vi "getPosInfo.vi"(11 "UI_DataIn":T2={"controlTabState"=[], "pathToSTLFiles"=path "", "availableObjs"=[], "objectNames"=[], "addedObjs"=[], "selectedObj"={"Name"="", "objectFiles"=[], "center"={"X"=0.0, "Y"=0.0, "Z"=0.0}, "extent"={"X"=0.0, "Y"=0.0, "Z"=0.0}, "allowedMotion"=enum."XY", "mountOn"=enum."yArm", "Movements"=[], "extraInfo"=[], "hasPOI?"=FALSE, "POI"={"X"=0.0, "Y"=0.0, "Z"=0.0}, "posOffset"={"X"=0.0, "Y"=0.0, "Z"=0.0}, "referenceNum"=refnum}, "3DPictureObjRef"=refnum, "yPOI_Home"={"X"=0.0, "Y"=0.0, "Z"=0.0}, "yPOI_Current"={"X"=0.0, "Y"=0.0, "Z"=0.0}, "yPOI_Added?"=FALSE, "homePos_Offset"={"X"=0.0, "Y"=0.0, "Z"=0.0}, "breadBoardOriginOffset"={"X"=25.4, "Y"=12.7, "Z"=12.7}, "XYtranslateObjControls"=[], "ZtranslateObjControls"=[], "pBot_controls"=[], "pBot_VISA"="", "commandLog"="", "pBotConnected?"=FALSE, "pBot_currentEEPROMsettings"="", "realTimeInfoControls"=[], "pBot_tempSensor1"=0.0, "pBot_tempSensor2"=0.0, "realTimeInfoTextColor"=[], "disconnectPBot_Event"=refnum, "needToHomeY?"=FALSE, "pBot_relativePositioning"=FALSE, "pBot_minPos"={"X"=0.0, "Y"=0.0, "Z"=0.0}, "pBot_maxPos"={"X"=0.0, "Y"=0.0, "Z"=0.0}, "pBot_homeOffset"={"X"=0.0, "Y"=0.0, "Z"=0.0}, "textColorGreen"=9174826, "textColorRed"=16750216, "textColorGray"=9868950, "transVisualizationControls"=[], "needToHomeXY?"=FALSE, "pBot_minScanRegion"={"X"=0.0, "Y"=0.0, "Z"=0.0}, "pBot_maxScanRegion"={"X"=0.0, "Y"=0.0, "Z"=0.0}, "pBot_scanN"={"X"=0, "Y"=0, "Z"=0}, "connectedInstruments"=[], "isScanning?"=FALSE, "Wavelengths"=[], "usb2000p_controlRefs"=[]}) -> (0 "hasPOI?":bool, 1 "POI":T1[](array[typedef]), 2 "extent":T1[](array[typedef]), 3 "origin":T1[](array[typedef]))   [LabVIEW 2015]
uses:
  controls/UI Data.ctl
  processedObjectInfo.ctl
  controls/scanInstrumentInfo.ctl
  <vilib>/Utility/miscctls.llb/LV3DPointTypeDef.ctl
  <userlib>/_MGI/Coordinates/MGI Apply Transform/MGI Apply Transform (DBL).vi
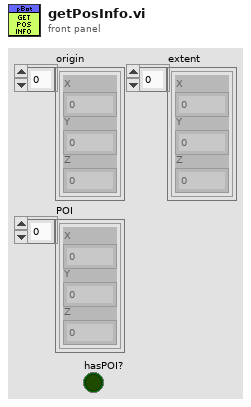
[diagram p1: front panel]
types:
  T1 = typedef "LV3DPointTypeDef.ctl" = cluster{"X":sgl, "Y":sgl, "Z":sgl}
  T2 = typedef "UI Data.ctl" = cluster{"controlTabState":bool[], "pathToSTLFiles":path, "availableObjs":T3[], "objectNames":string[], "addedObjs":T3[], "selectedObj":T3, "3DPictureObjRef":refnum<vi>, "yPOI_Home":cluster{"X":dbl, "Y":dbl, "Z":dbl}, "yPOI_Current":cluster{"X":dbl, "Y":dbl, "Z":dbl}, "yPOI_Added?":bool, "homePos_Offset":cluster{"X":dbl, "Y":dbl, "Z":dbl}, "breadBoardOriginOffset":cluster{"X":dbl, "Y":dbl, "Z":dbl}, "XYtranslateObjControls":refnum<vi>[], "ZtranslateObjControls":refnum<vi>[], "pBot_controls":refnum<vi>[], "pBot_VISA":refnum<visa-resource-name>, "commandLog":string, "pBotConnected?":bool, "pBot_currentEEPROMsettings":string, "realTimeInfoControls":refnum<vi>[], "pBot_tempSensor1":dbl, "pBot_tempSensor2":dbl, "realTimeInfoTextColor":u32[], "disconnectPBot_Event":refnum<user-event>, "needToHomeY?":bool, "pBot_relativePositioning":bool, "pBot_minPos":cluster{"X":dbl, "Y":dbl, "Z":dbl}, "pBot_maxPos":cluster{"X":dbl, "Y":dbl, "Z":dbl}, "pBot_homeOffset":cluster{"X":dbl, "Y":dbl, "Z":dbl}, "textColorGreen":u32, "textColorRed":u32, "textColorGray":u32, "transVisualizationControls":refnum<vi>[], "needToHomeXY?":bool, "pBot_minScanRegion":cluster{"X":sgl, "Y":sgl, "Z":sgl}, "pBot_maxScanRegion":cluster{"X":sgl, "Y":sgl, "Z":sgl}, "pBot_scanN":cluster{"X":u16, "Y":u16, "Z":u16}, "connectedInstruments":T4[], "isScanning?":bool, "Wavelengths":dbl[], "usb2000p_controlRefs":refnum<vi>[]}
  T3 = typedef "processedObjectInfo.ctl" = cluster{"Name":string, "objectFiles":cluster{"Location":path, "Color":cluster{"R":dbl, "G":dbl, "B":dbl, "A":dbl}}[], "center":cluster{"X":dbl, "Y":dbl, "Z":dbl}, "extent":cluster{"X":dbl, "Y":dbl, "Z":dbl}, "allowedMotion":enum16{"XY", "Z"}, "mountOn":enum16{"yArm", "breadBoard"}, "Movements":cluster{"Type":enum16{"rr", "ra", "tr", "ta"}, "vector":cluster{"X":dbl, "Y":dbl, "Z":dbl}, "scalar":dbl}[], "extraInfo":cluster{"parameter":string, "dataType":string, "vector":cluster{"X":dbl, "Y":dbl, "Z":dbl}, "scalar":dbl}[], "hasPOI?":bool, "POI":cluster{"X":dbl, "Y":dbl, "Z":dbl}, "posOffset":cluster{"X":dbl, "Y":dbl, "Z":dbl}, "referenceNum":refnum<vi>}
  T4 = typedef "scanInstrumentInfo.ctl" = cluster{"Name":string, "VISAname":refnum<visa-resource-name>, "1D_dataArraySize":u16, "extraInfo":variant, "error":errorcluster}
  T5 = cluster{"yPOI_Current":cluster{"X":dbl, "Y":dbl, "Z":dbl}, "yPOI_Home":cluster{"X":dbl, "Y":dbl, "Z":dbl}, "breadBoardOriginOffset":cluster{"X":dbl, "Y":dbl, "Z":dbl}, "homePos_Offset":cluster{"X":dbl, "Y":dbl, "Z":dbl}}
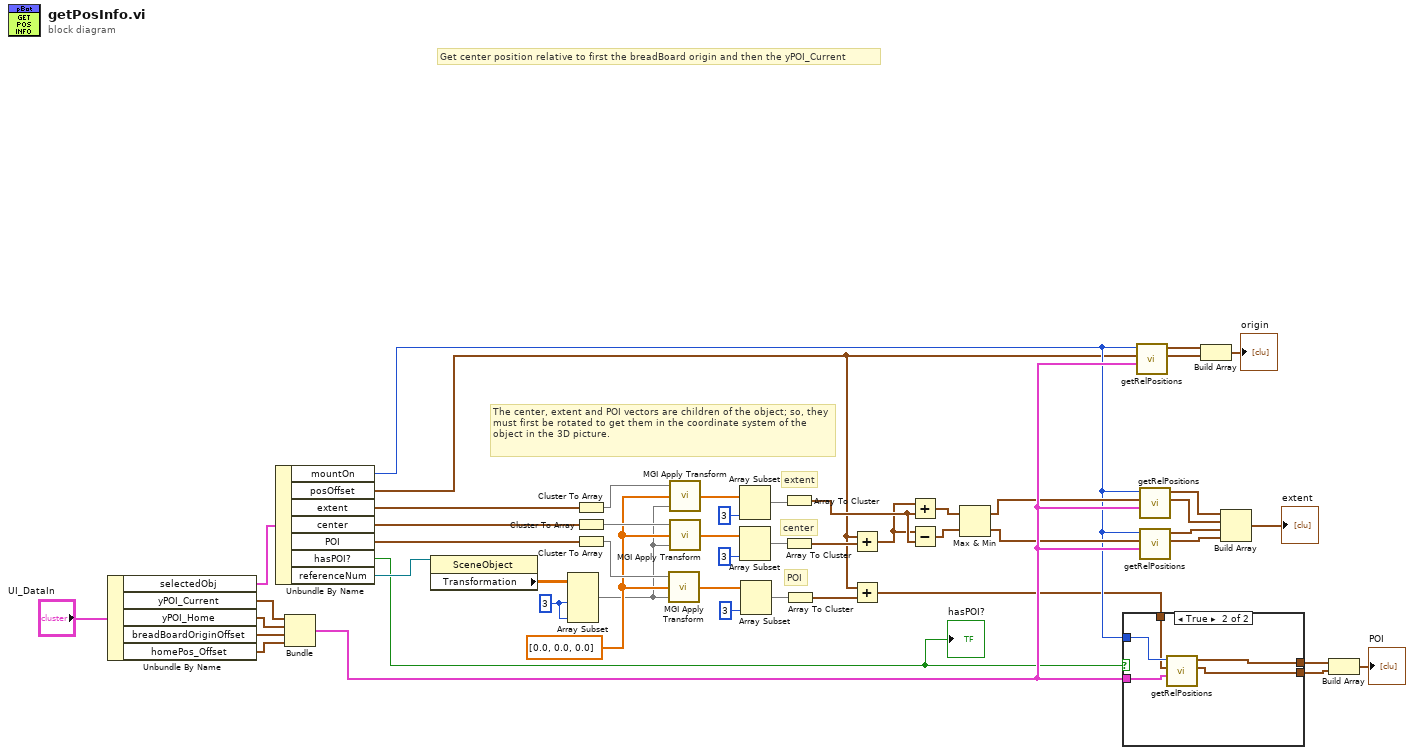
[diagram p0: block diagram]
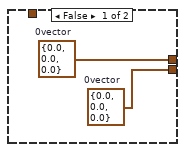
[diagram p2: hidden frame]
diagram:
  w25 = sgl[] [0.0, 0.0, 0.0] ("Origin Vector")
  w41 = 3 ("length")
  # "POI"
  # "center"
  # "extent"
  # "The center, extent and POI vectors are children of the object; so, they must first be rotated to get them in the coordinate system of the object in the 3D picture."
  # "Get center position relative to first the breadBoard origin and then the yPOI_Current"
  n1 = Unbundle By Name("UI_DataIn") -> ("selectedObj"=w50:T3, "yPOI_Current"=w19:cluster{"X":dbl, "Y":dbl, "Z":dbl}, "yPOI_Home"=w18:cluster{"X":dbl, "Y":dbl, "Z":dbl}, "breadBoardOriginOffset"=w17:cluster{"X":dbl, "Y":dbl, "Z":dbl}, "homePos_Offset"=w16:cluster{"X":dbl, "Y":dbl, "Z":dbl})
  n2 = Unbundle By Name(w50) -> ("mountOn"=w12:enum16{"yArm", "breadBoard"}, "posOffset"=w2:cluster{"X":dbl, "Y":dbl, "Z":dbl}, "extent"=w22:cluster{"X":dbl, "Y":dbl, "Z":dbl}, "center"=w21:cluster{"X":dbl, "Y":dbl, "Z":dbl}, "POI"=w7:cluster{"X":dbl, "Y":dbl, "Z":dbl}, "hasPOI?"=w6:bool, "referenceNum"=w43:refnum<vi>)
  "hasPOI?" <- w6
  n3 = Bundle("yPOI_Current"=w19, "yPOI_Home"=w18, "breadBoardOriginOffset"=w17, "homePos_Offset"=w16) -> (w15:T5)  [unwired: 1 in]
  n4 = property class="SceneObject"(reference=w43) -> ("Transformation"=w42:sgl[][])  [unwired: 1 in, 2 out]
  n5 = Array Subset(array=w42, length (row)=w41, length (col)=w41) -> (w24:sgl[][])  [unwired: 2 in]
  n6 = Cluster To Array(cluster=w22) -> (array=w23:dbl[])
  n7 = Cluster To Array(cluster=w21) -> (array=w29:dbl[])
  n8 = Cluster To Array(cluster=w7) -> (array=w40:dbl[])
  n9 = call-poly <userlib>:"MGI Apply Transform.vi"("Rotation Matrix"=w24, "Origin Vector"=w25, "Raw Vector"=w40) -> ("Transformed Vector"=w39:dbl[])
  n10 = call-poly <userlib>:"MGI Apply Transform.vi"("Rotation Matrix"=w24, "Origin Vector"=w25, "Raw Vector"=w23) -> ("Transformed Vector"=w28:dbl[])
  n11 = call-poly <userlib>:"MGI Apply Transform.vi"("Rotation Matrix"=w24, "Origin Vector"=w25, "Raw Vector"=w29) -> ("Transformed Vector"=w30:dbl[])
  n12 = Array Subset(array=w28, length=3) -> (w26:dbl[])  [unwired: 1 in]
  n13 = Array Subset(array=w30, length=3) -> (w32:dbl[])  [unwired: 1 in]
  n14 = Array Subset(array=w39, length=3) -> (w37:dbl[])  [unwired: 1 in]
  n15 = Array To Cluster(array=w26) -> (cluster=w20:cluster{"[0]":dbl, "[1]":dbl, "[2]":dbl})
  n16 = Array To Cluster(array=w32) -> (cluster=w5:cluster{"[0]":dbl, "[1]":dbl, "[2]":dbl})
  n17 = Array To Cluster(array=w37) -> (cluster=w3:cluster{"[0]":dbl, "[1]":dbl, "[2]":dbl})
  n18 = Add(x=w2, y=w5) -> (x+y=w4:cluster{dbl, dbl, dbl})
  n19 = Add(x=w2, y=w3) -> (x+y=w1:cluster{dbl, dbl, dbl})
  n20 = Add(x=w4, y=w20) -> (x+y=w34:cluster{dbl, dbl, dbl})
  n21 = Subtract(x=w4, y=w20) -> (x-y=w33:cluster{dbl, dbl, dbl})
  n22 = Max & Min(x=w34, y=w33) -> (max(x,y)=w13:cluster{dbl, dbl, dbl}, min(x,y)=w14:cluster{dbl, dbl, dbl})
  n23 = case shown="True" w6 {
    tunnel: w12 -> [_ w57]
    tunnel: [w52 w56] -> w47
    tunnel: [w51 w55] -> w46
    tunnel: w15 -> [_ w54]
    tunnel: w1 -> [_ w53]
    frame False {
      w51 = T1 {"X"=0.0, "Y"=0.0, "Z"=0.0}  # 0vector
      w52 = T1 {"X"=0.0, "Y"=0.0, "Z"=0.0}  # 0vector
    }
    frame True {
      n24 = call "getRelPositions.vi"("originOffsetVectors"=w54, "point"=w53, "mountOn"=w57) -> ("to_yPOI"=w55:T1, "to_BBorigin"=w56:T1)  [unwired: 7 in]
    }
  }
  n25 = call "getRelPositions.vi"("originOffsetVectors"=w15, "point"=w2, "mountOn"=w12) -> ("to_yPOI"=w35:T1, "to_BBorigin"=w36:T1)  [unwired: 7 in]
  n26 = call "getRelPositions.vi"("originOffsetVectors"=w15, "point"=w13, "mountOn"=w12) -> ("to_yPOI"=w11:T1, "to_BBorigin"=w10:T1)  [unwired: 7 in]
  n27 = call "getRelPositions.vi"("originOffsetVectors"=w15, "point"=w14, "mountOn"=w12) -> ("to_yPOI"=w8:T1, "to_BBorigin"=w9:T1)  [unwired: 7 in]
  n28 = Build Array(w36, w35) -> (→"origin":T1[])
  n29 = Build Array(w10, w11, w9, w8) -> (→"extent":T1[])
  n30 = Build Array(w47, w46) -> (→"POI":T1[])
